vi "Wait.Gui.Open.vi"(8 "error in (no error)":errorcluster, 9 "ProgBarSize (0)":i32, 10 "Status (\"\")":string, 11 "Msg":string) -> (0 "error out":errorcluster)   [LabVIEW 2016]
uses:
  Wait.Gui.Action.ctl
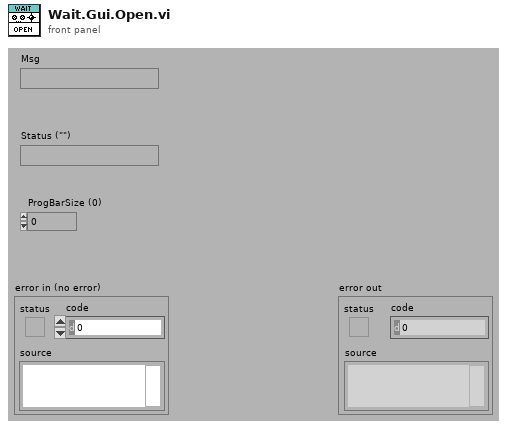
[diagram p1: front panel]
types:
  T1 = typedef "Wait.Gui.Action.ctl" = enum32{"idle", "constructor", "destructor", "--- GuiServerWait ---", "open FP", "close FP", "update msg", "update progbar"}
  T2 = cluster{"Msg":string, "Status (\"\")":string, "ProgBarSize (0)":i32}
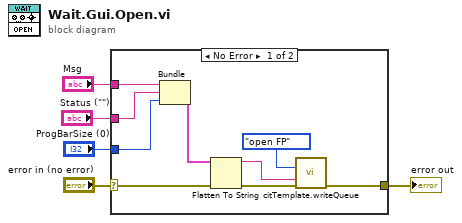
[diagram p0: block diagram]
diagram:
  n1 = case shown="No Error" "error in (no error)" {
    selector: "error in (no error)" -> [w6 w15]
    tunnel: [w14 w15] -> w5
    tunnel: "Msg" -> [w10 _]
    tunnel: "Status (\"\")" -> [w9 _]
    tunnel: "ProgBarSize (0)" -> [w8 _]
    frame No Error {
      n2 = Bundle("Msg"=w10, "Status (\"\")"=w9, "ProgBarSize (0)"=w8) -> (w7:T2)  [unwired: 1 in]
      n3 = Flatten To String(anything=w7, error in (no error)=w6) -> (data string=w12:string, error out=w11:errorcluster)  [unwired: 2 in, 1 out]
      n4 = call "citTemplate.writeQueue.vi"("event in (if not connected:all statemachine with data event)"=Wait.Gui.Action."open FP" ("Action"), "data in"=w12, "error in (no error)"=w11) -> ("error out"=w14:errorcluster)  [unwired: 12 in]
    }
    frame Error {
    }
  }
  "error out" <- w5
